vi "SDCP - Standard Message Frame - Parameter Encode & Decode Test.vi"() -> ()   [LabVIEW 2020]
uses:
  Typedefs/SDCP - SMF parameter descriptors.ctl
  Typedefs/SDCP - Standard Message Frames FGV - Commands.ctl
  Typedefs/SDCP - Standard Message Frame Parameters - FGV - commands.ctl
panel:
  in  "index 2":i32
  in  "index 1":i32
  out "SMF Parameters out 2":T1[](array[typedef])
  out "Encoded message frame 2":u8[](array[numeric])
  in  "Value in 2":string
  out "SMF Parameters out 1":T1[](array[typedef])
  out "Encoded message frame 1":u8[](array[numeric])
  in  "Value in 1":string
  out "SMF Parameters descriptors out":T1[](array[typedef])
  in  "Parameter file path":path
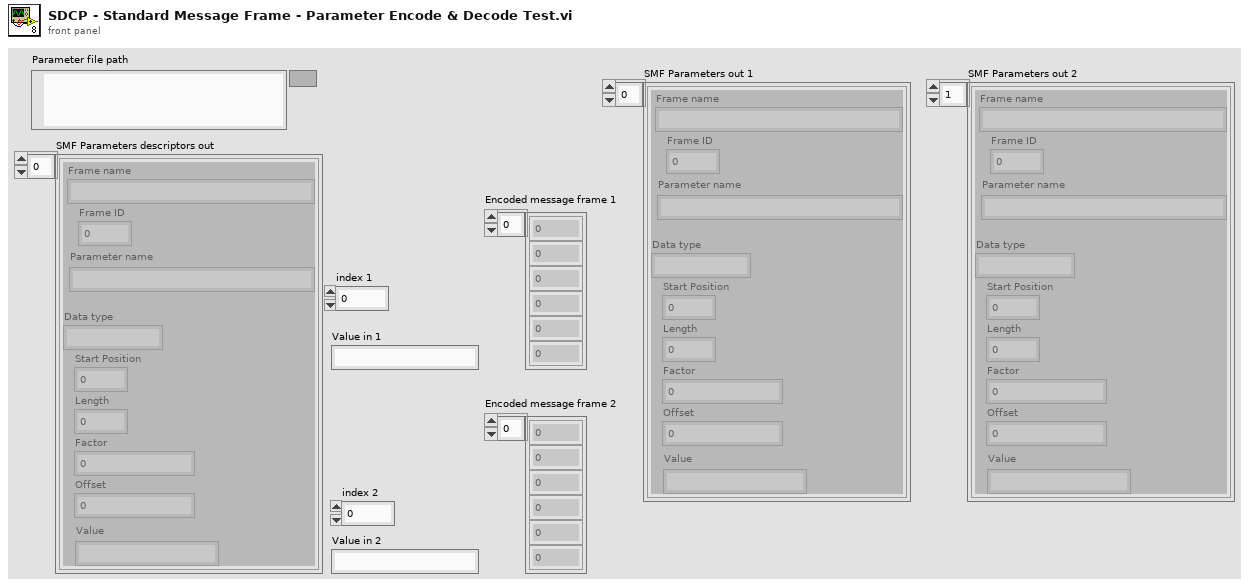
[diagram p1: front panel]
types:
  T1 = typedef "SDCP - SMF parameter descriptors.ctl" = cluster{"Frame name":string, "Frame ID":i32, "Data type":string, "Start Position":i32, "Length":i32, "Factor":dbl, "Offset":dbl, "Parameter name":string, "Value":string}
  T2 = typedef "SDCP - Standard Message Frame Parameters - FGV - commands.ctl" = enum16{"Write descriptors", "Read descriptors", "Read values", "Load parameters from file", "Write values"}
  T3 = typedef "SDCP - Standard Message Frames FGV - Commands.ctl" = enum16{"Reset", "Read", "Write", "Set Priority"}
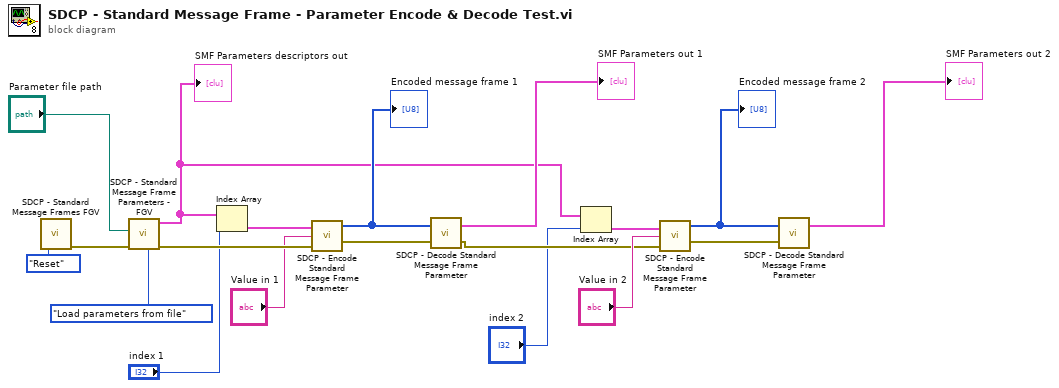
[diagram p0: block diagram]
diagram:
  n1 = call "SDCP - Standard Message Frames FGV.vi"("Command"=SDCP_-_Standard_Message_Frames_FGV_-_Commands."Reset") -> ("error out"=w18:errorcluster)  [unwired: 5 in, 2 out]
  n2 = call "SDCP - Standard Message Frame Parameters - FGV.vi"("Parameter file path"="Parameter file path", "error in (no error)"=w18, "Command"=SDCP_-_Standard_Message_Frame_Parameters_-_FGV_-_commands."Load parameters from file") -> ("SMF Parameters descriptors out"=w3:T1[], "error out"=w15:errorcluster)  [unwired: 4 in]
  "SMF Parameters descriptors out" <- w3
  n3 = Index Array(array=w3, index="index 1") -> (element=w13:T1)
  n4 = call "SDCP - Encode Standard Message Frame Parameter.vi"("error in (no error)"=w15, "Value in"="Value in 1", "SMF descriptor in"=w13) -> ("error out"=w11:errorcluster, "Encoded message frame"=w10:u8[])  [unwired: 1 in]
  "Encoded message frame 1" <- w10
  n5 = call "SDCP - Decode Standard Message Frame Parameter.vi"("error in (no error)"=w11, "Bytes in"=w10) -> ("error out"=w4:errorcluster, "SMF Parameters out"=→"SMF Parameters out 1":T1[])
  n6 = Index Array(array=w3, index="index 2") -> (element=w2:T1)
  n7 = call "SDCP - Encode Standard Message Frame Parameter.vi"("error in (no error)"=w4, "Value in"="Value in 2", "SMF descriptor in"=w2) -> ("error out"=w7:errorcluster, "Encoded message frame"=w6:u8[])  [unwired: 1 in]
  "Encoded message frame 2" <- w6
  n8 = call "SDCP - Decode Standard Message Frame Parameter.vi"("error in (no error)"=w7, "Bytes in"=w6) -> ("SMF Parameters out"=→"SMF Parameters out 2":T1[])  [unwired: 1 out]
